vi "Read Array Key (Raw).vi"(7 "Section Name":string, 8 "error in (no error)":errorcluster, 10 "Key Name":string, 11 "Config in":refnum<class "LabVIEW-Config.lvclass">) -> (0 "error out":errorcluster, 1 "Content":string[](array[string]), 2 "Key Found?":bool, 3 "Config out":refnum<class "LabVIEW-Config.lvclass">)   [LabVIEW 2017, in "LabVIEW-Config.lvlib" / "LabVIEW-Config.lvclass"]
uses:
  LabVIEW-Config.lvclass
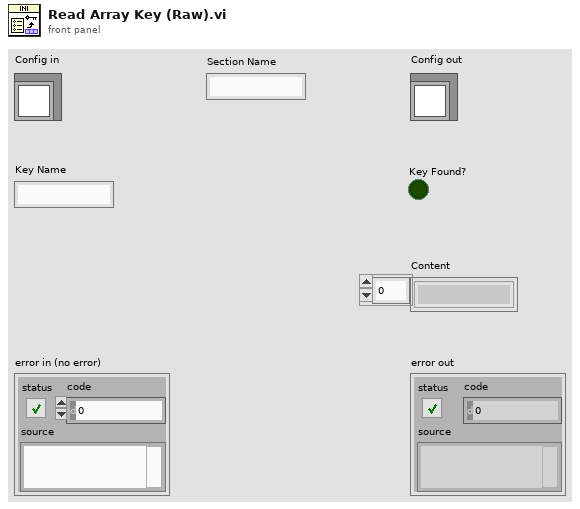
[diagram p1: front panel]
types:
  T1 = typedef "LabVIEW-Config.lvlib/LabVIEW-Config.lvclass/LineToken.ctl" = enum8{"comment", "section", "key", "more"}
  T2 = typedef "LabVIEW-Config.lvlib/LabVIEW-Config.lvclass/KeyInfo.ctl" = cluster{"Key Indexes":cluster{"Indexes":i32[]}[], "Session Found?":bool, "Key found?":bool, "Session Index":i32}
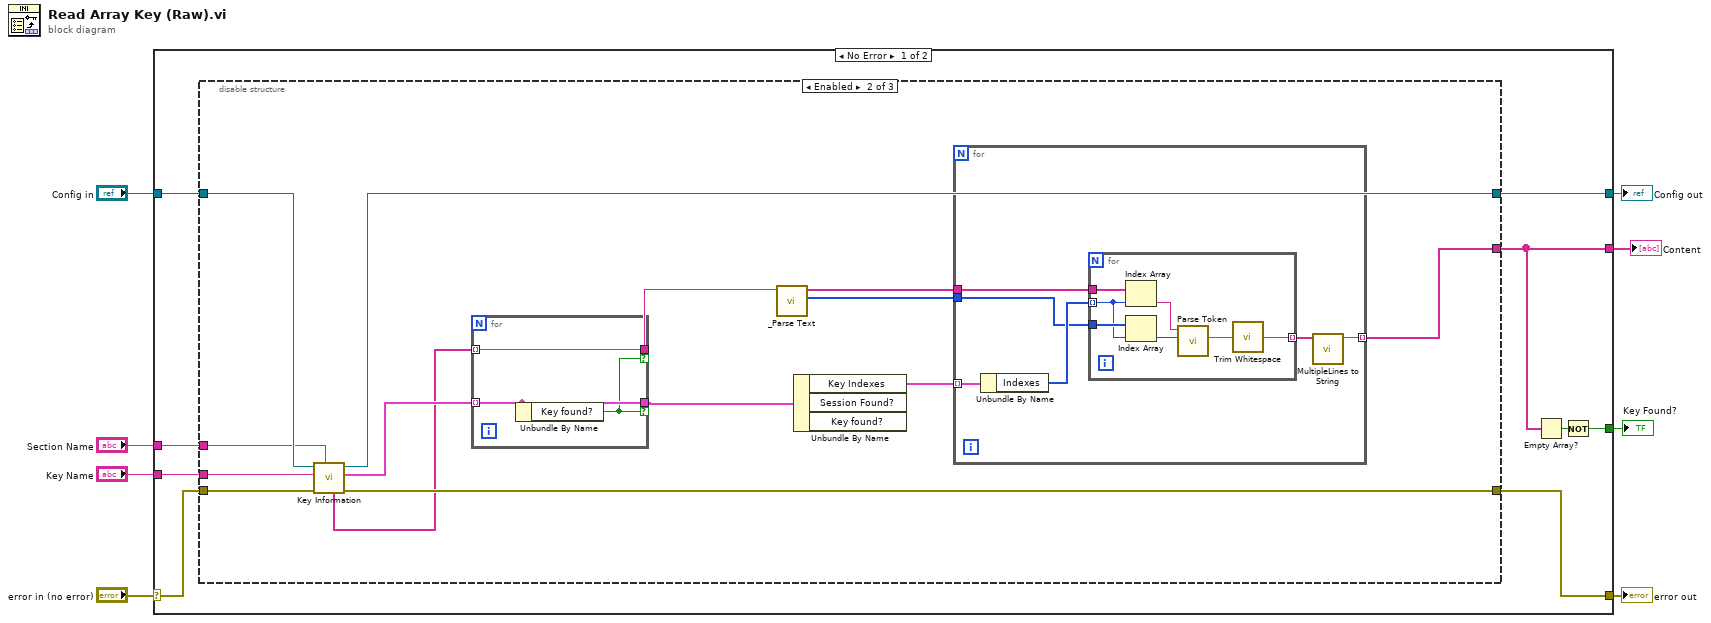
[diagram p0: block diagram]
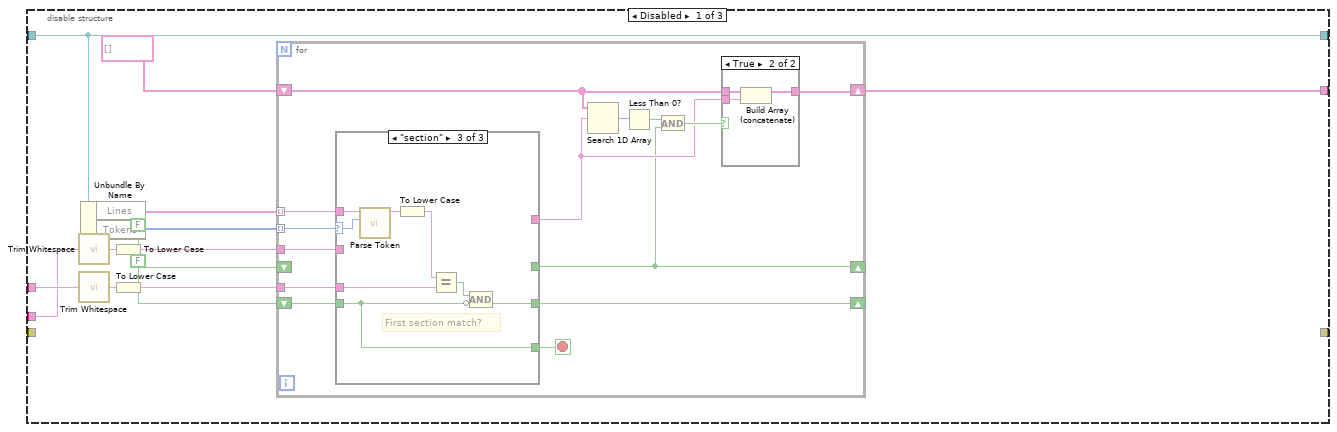
[diagram p2: hidden frame]
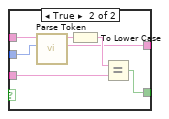
[diagram p6: hidden frame]
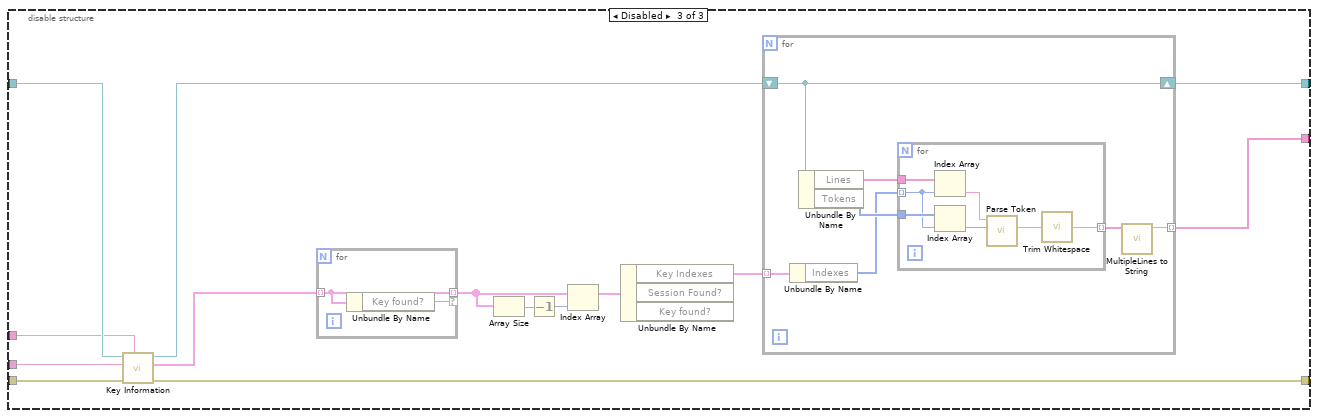
[diagram p7: hidden frame]
diagram:
  n1 = case shown="No Error" "error in (no error)" {
    selector: "error in (no error)" -> [w10 w132]
    tunnel: "Config in" -> [w16 w131]
    tunnel: [w9 w132] -> w7
    tunnel: [w11 w131] -> w5
    tunnel: "Section Name" -> [w17 _]
    tunnel: "Key Name" -> [w15 _]
    tunnel: [w14 _] -> w2
    tunnel: [w12 _] -> w1
    frame No Error {
      n2 = disable-structure shown="Enabled" {
        disable-tunnel: w17 -> [w29 w83 w113]
        disable-tunnel: w16 -> [w18 w84 w114]
        disable-tunnel: w15 -> [w25 w82 w112]
        disable-tunnel: [w21 w77 w101] -> w14
        disable-tunnel: [w18 w74 w102] -> w11
        disable-tunnel: w10 -> [_ w81 w111]
        disable-tunnel: [_ w80 w110] -> w9
        frame Disabled {
          n3 = call <vilib>:"Trim Whitespace.vi"("string"=w25) -> ("trimmed string"=w19:string)  [unwired: 1 in]
          n4 = call <vilib>:"Trim Whitespace.vi"("string"=w29) -> ("trimmed string"=w20:string)  [unwired: 1 in]
          n5 = Unbundle By Name(w18) -> ("Lines"=w30:string[], "Tokens"=w23:T1[])
          n6 = To Lower Case(string=w19) -> (all lower case string=w24:string)
          n7 = To Lower Case(string=w20) -> (all lower case string=w28:string)
          n8 = for {
            tunnel: w23 -> [w44] mode=indexing
            tunnel: w30 -> [w43] mode=indexing
            tunnel: w28 -> [w42]
            shift-right: [w40] -> _
            shift-left: FALSE -> [w41]
            shift-right: [w32] -> _
            shift-left: FALSE -> [_]
            tunnel: w24 -> [w39]
            shift-right: [w35] -> w21
            shift-left: string[] [] -> [w34]
            stop <- w31 stop-if-true
            n9 = case shown="\"section\"" w44 {
              selector: w44 -> [_ w50 w65]
              tunnel: w43 -> [_ w55 w66]
              tunnel: w42 -> [_ _ w70]
              tunnel: [w49 w54 w67] -> w40
              tunnel: w41 -> [w49 w54 w63]
              tunnel: w39 -> [_ w53 _]
              tunnel: [_ w52 _] -> w32
              tunnel: [_ w51 _] -> w33
              tunnel: [_ _ w63] -> w31
              frame "comment", "more" {
              }
              frame "key" {
                n10 = case "Key in Section?" shown="False" w54 {
                  tunnel: w55 -> [_ w59]
                  tunnel: w53 -> [_ w62]
                  tunnel: [_ w60] -> w52
                  tunnel: [_ w56] -> w51
                  tunnel: w50 -> [_ w58]
                  frame False {
                  }
                  frame True {
                    n11 = call "Parse Token.vi"("Token"=w58, "Line"=w59) -> ("Value"=w56:string, "Name"=w57:string)  [unwired: 8 in]
                    n12 = To Lower Case(string=w57) -> (all lower case string=w61:string)
                    n13 = Equal?(x=w61, y=w62) -> (x = y?=w60:bool)
                  }
                }
              }
              frame "section" {
                # "First section match?"
                n14 = call "Parse Token.vi"("Token"=w65, "Line"=w66) -> ("Name"=w64:string)  [unwired: 8 in, 1 out]
                n15 = To Lower Case(string=w64) -> (all lower case string=w69:string)
                n16 = Equal?(x=w69, y=w70) -> (x = y?=w68:bool)
                n17 = Compound Arithmetic op=AND(w68, invert w63) -> (w67:bool)
              }
            }
            n18 = Search 1D Array(1D array=w34, element=w33) -> (index of element=w38:i32)  [unwired: 1 in]
            n19 = Less Than 0?(x=w38) -> (x < 0?=w37:bool)
            n20 = And(x=w37, y=w32) -> (x .and. y?=w36:bool)
            n21 = case shown="True" w36 {
              tunnel: [w45 w48] -> w35
              tunnel: w34 -> [w45 w47]
              tunnel: w33 -> [_ w46]
              frame False {
              }
              frame True {
                n22 = Build Array (concatenate)(w47, w46) -> (w48:string[])
              }
            }
          }
        }
        frame Enabled {
          n23 = call "Key Information.vi"("Section Name"=w83, "error in (no error)"=w81, "Key Name"=w82, "Config in"=w84) -> ("error out"=w80:errorcluster, "Key Information"=w78:T2[], "Config out"=w74:refnum<class "LabVIEW-Config.lvclass">, "Section Content"=w76:string[])  [unwired: 3 in, 1 out]
          n24 = for {
            tunnel: w78 -> [w100] mode=indexing
            tunnel: [w100] -> w75 if=w98
            tunnel: w76 -> [w99] mode=indexing
            tunnel: [w99] -> w73 if=w98
            n25 = Unbundle By Name(w100) -> ("Key found?"=w98:bool)
          }
          n26 = call "_Parse Text.vi"("Text"=w73) -> ("Tokens"=w72:T1[], "Lines"=w71:string[])  [unwired: 9 in]
          n27 = Unbundle By Name(w75) -> ("Key Indexes"=w79:cluster{"Indexes":i32[]}[])  [unwired: 2 out]
          n28 = for {
            tunnel: w79 -> [w89] mode=indexing
            tunnel: [w87] -> w77 mode=indexing
            tunnel: w71 -> [w86]
            tunnel: w72 -> [w85]
            n29 = Unbundle By Name(w89) -> ("Indexes"=w88:i32[])
            n30 = for {
              tunnel: w86 -> [w97]
              tunnel: w88 -> [w94] mode=indexing
              tunnel: w85 -> [w95]
              tunnel: [w91] -> w90 mode=indexing
              n31 = Index Array(array=w97, index=w94) -> (element=w96:string)
              n32 = Index Array(array=w95, index=w94) -> (element=w93:T1)
              n33 = call "Parse Token.vi"("Token"=w93, "Line"=w96) -> ("Value"=w92:string)  [unwired: 8 in, 1 out]
              n34 = call <vilib>:"Trim Whitespace.vi"("string"=w92) -> ("trimmed string"=w91:string)  [unwired: 1 in]
            }
            n35 = call "MultipleLines to String.vi"("Array"=w90) -> ("String"=w87:string)  [unwired: 10 in]
          }
        }
        frame Disabled {
          n36 = call "Key Information.vi"("Section Name"=w113, "error in (no error)"=w111, "Key Name"=w112, "Config in"=w114) -> ("error out"=w110:errorcluster, "Key Information"=w104:T2[], "Config out"=w103:refnum<class "LabVIEW-Config.lvclass">)  [unwired: 3 in, 2 out]
          n37 = for {
            tunnel: w104 -> [w130] mode=indexing
            tunnel: [w130] -> w105 mode=indexing if=w129
            n38 = Unbundle By Name(w130) -> ("Key found?"=w129:bool)
          }
          n39 = Array Size(array=w105) -> (size(s)=w107:i32)
          n40 = Decrement(x=w107) -> (x-1=w106:i32)
          n41 = Index Array(array=w105, index=w106) -> (element=w108:T2)
          n42 = Unbundle By Name(w108) -> ("Key Indexes"=w109:cluster{"Indexes":i32[]}[])  [unwired: 2 out]
          n43 = for {
            tunnel: w109 -> [w118] mode=indexing
            shift-right: [w116] -> w102
            shift-left: w103 -> [w116]
            tunnel: [w115] -> w101 mode=indexing
            n44 = Unbundle By Name(w118) -> ("Indexes"=w117:i32[])
            n45 = Unbundle By Name(w116) -> ("Lines"=w121:string[], "Tokens"=w120:T1[])
            n46 = for {
              tunnel: w121 -> [w128]
              tunnel: w117 -> [w125] mode=indexing
              tunnel: w120 -> [w126]
              tunnel: [w122] -> w119 mode=indexing
              n47 = Index Array(array=w128, index=w125) -> (element=w127:string)
              n48 = Index Array(array=w126, index=w125) -> (element=w124:T1)
              n49 = call "Parse Token.vi"("Token"=w124, "Line"=w127) -> ("Value"=w123:string)  [unwired: 8 in, 1 out]
              n50 = call <vilib>:"Trim Whitespace.vi"("string"=w123) -> ("trimmed string"=w122:string)  [unwired: 1 in]
            }
            n51 = call "MultipleLines to String.vi"("Array"=w119) -> ("String"=w115:string)  [unwired: 10 in]
          }
        }
      }
      n52 = Empty Array?(array=w14) -> (empty?=w13:bool)
      n53 = Not(x=w13) -> (.not. x?=w12:bool)
    }
    frame Error {
    }
  }
  "error out" <- w7
  "Config out" <- w5
  "Content" <- w2
  "Key Found?" <- w1
